vi "Sousvi2.vi"(0 "Combo Box 2":string(combo), 1 "Coffee extraction":bool) -> (2 "subarray":string[](array[string]), 3 "Numeric":i32, 4 "Array":bool[][](array[boolean]))   [LabVIEW 2022 SP3]
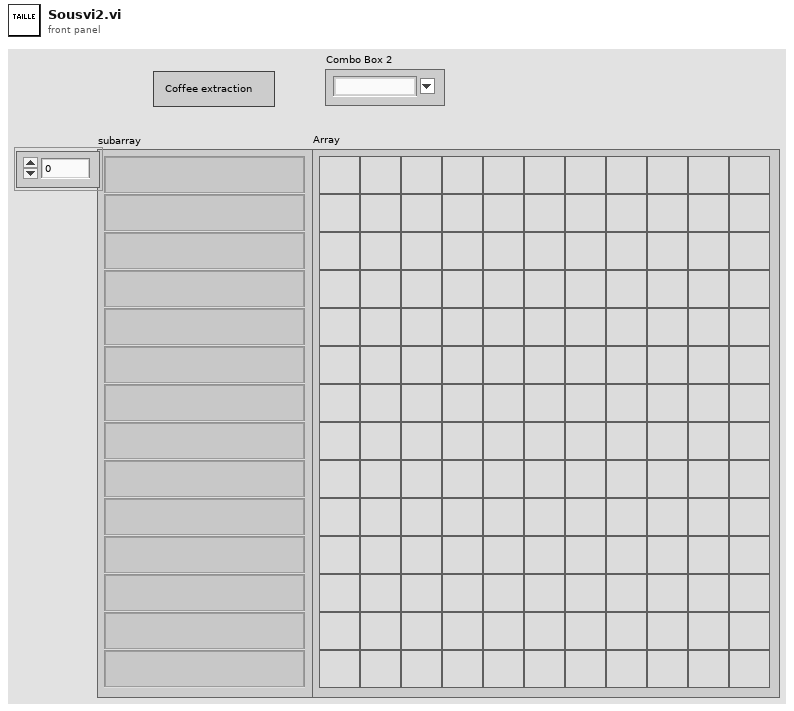
[diagram p1: front panel]
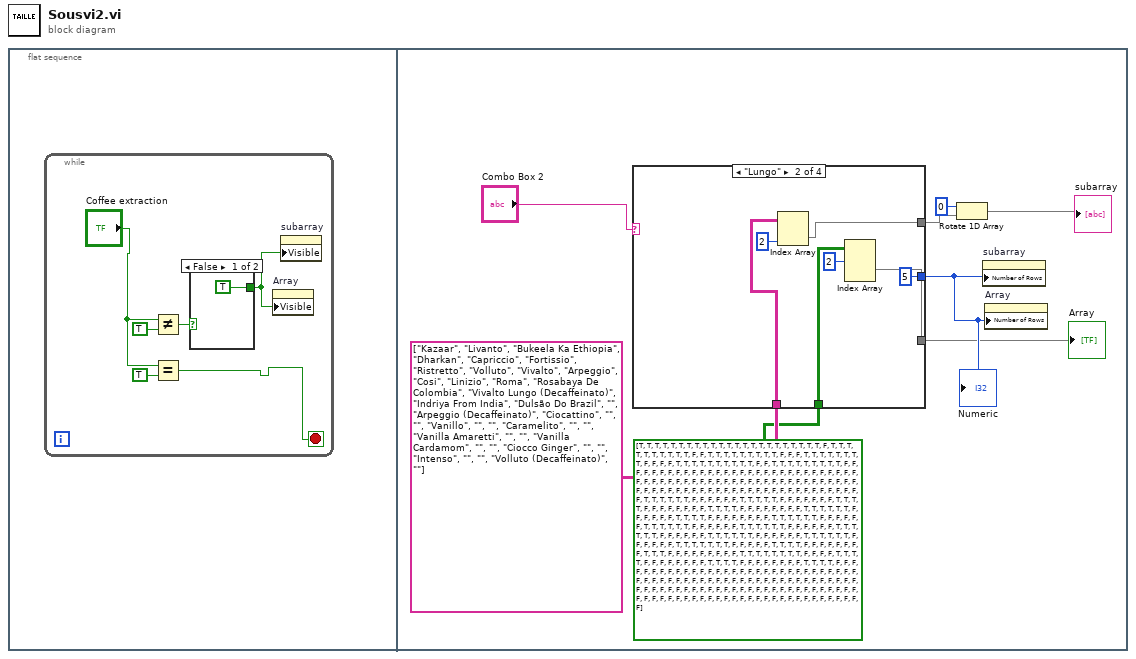
[diagram p0: block diagram]
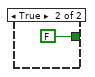
[diagram p2: hidden frame]
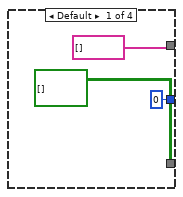
[diagram p3: hidden frame]
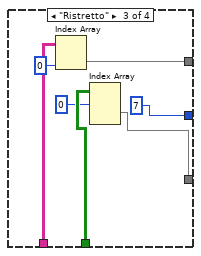
[diagram p4: hidden frame]
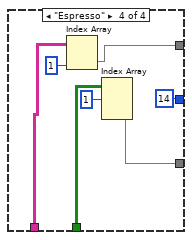
[diagram p5: hidden frame]
diagram:
  n1 = flat-sequence {
    frame #0 {
      n2 = while {
        stop <- w1 stop-if-true
        n3 = Not Equal?(x="Coffee extraction", y=TRUE) -> (x != y?=w5:bool)
        n4 = Equal?(x="Coffee extraction", y=TRUE) -> (x = y?=w1:bool)
        n5 = case shown="False" w5 {
          tunnel: [TRUE FALSE] -> w2
          frame False {
          }
          frame True {
          }
        }
        n6 = property on="Array" class="Arr (strict)"("Visible"=w2) -> ()  [unwired: 2 in, 2 out]
        n7 = property on="subarray" class="Arr (strict)"("Visible"=w2) -> ()  [unwired: 2 in, 2 out]
      }
    }
    frame #1 {
      n8 = case shown="\"Lungo\"" "Combo Box 2" {
        tunnel: string[][] [["Kazaar", "Livanto", "Bukeela Ka Ethiopia"], ["Dharkan", "Capriccio", "Fortissio"], ["Ristretto", "Volluto", "Vivalto"], ["Arpeggio", "Cosi", "Linizio"], ["Roma", "Rosabaya De Colombia", "Vivalto Lungo (Decaffeinato)"], ["Indriya From India", "Dulsão Do Brazil", ""], ["Arpeggio (Decaffeinato)", "Ciocattino", ""], ["", "Vanillo", ""], ["", "Caramelito", ""], ["", "Vanilla Amaretti", ""], ["", "Vanilla Cardamom", ""], ["", "Ciocco Ginger", ""], ["", "Intenso", ""], ["", "Volluto (Decaffeinato)", ""]] -> [_ w25 w33 w38]
        tunnel: [string[] [] ("subarray") w24 w31 w39] -> w13
        tunnel: [0 5 7 14] -> w16
        tunnel: bool[][][] [[[TRUE, TRUE, TRUE, TRUE, TRUE, TRUE, TRUE, TRUE, TRUE, TRUE, TRUE, TRUE], [TRUE, TRUE, TRUE, TRUE, TRUE, TRUE, TRUE, TRUE, TRUE, TRUE, TRUE, FALSE], [TRUE, TRUE, TRUE, TRUE, TRUE, TRUE, TRUE, TRUE, TRUE, TRUE, FALSE, FALSE], [TRUE, TRUE, TRUE, TRUE, TRUE, TRUE, TRUE, TRUE, TRUE, FALSE, FALSE, FALSE], [TRUE, TRUE, TRUE, TRUE, TRUE, TRUE, TRUE, TRUE, FALSE, FALSE, FALSE, FALSE], [TRUE, TRUE, TRUE, TRUE, TRUE, TRUE, TRUE, TRUE, TRUE, TRUE, FALSE, FALSE], [TRUE, TRUE, TRUE, TRUE, TRUE, TRUE, TRUE, TRUE, TRUE, FALSE, FALSE, FALSE], [FALSE, FALSE, FALSE, FALSE, FALSE, FALSE, FALSE, FALSE, FALSE, FALSE, FALSE, FALSE], [FALSE, FALSE, FALSE, FALSE, FALSE, FALSE, FALSE, FALSE, FALSE, FALSE, FALSE, FALSE], [FALSE, FALSE, FALSE, FALSE, FALSE, FALSE, FALSE, FALSE, FALSE, FALSE, FALSE, FALSE], [FALSE, FALSE, FALSE, FALSE, FALSE, FALSE, FALSE, FALSE, FALSE, FALSE, FALSE, FALSE], [FALSE, FALSE, FALSE, FALSE, FALSE, FALSE, FALSE, FALSE, FALSE, FALSE, FALSE, FALSE], [FALSE, FALSE, FALSE, FALSE, FALSE, FALSE, FALSE, FALSE, FALSE, FALSE, FALSE, FALSE], [FALSE, FALSE, FALSE, FALSE, FALSE, FALSE, FALSE, FALSE, FALSE, FALSE, FALSE, FALSE]], [[TRUE, TRUE, TRUE, TRUE, TRUE, TRUE, FALSE, FALSE, FALSE, FALSE, FALSE, FALSE], [TRUE, TRUE, TRUE, TRUE, TRUE, FALSE, FALSE, FALSE, FALSE, FALSE, FALSE, FALSE], [TRUE, TRUE, TRUE, TRUE, FALSE, FALSE, FALSE, FALSE, FALSE, FALSE, FALSE, FALSE], [TRUE, TRUE, TRUE, TRUE, FALSE, FALSE, FALSE, FALSE, FALSE, FALSE, FALSE, FALSE], [TRUE, TRUE, TRUE, TRUE, TRUE, TRUE, FALSE, FALSE, FALSE, FALSE, FALSE, FALSE], [TRUE, TRUE, TRUE, TRUE, FALSE, FALSE, FALSE, FALSE, FALSE, FALSE, FALSE, FALSE], [TRUE, TRUE, TRUE, TRUE, TRUE, TRUE, FALSE, FALSE, FALSE, FALSE, FALSE, FALSE], [TRUE, TRUE, TRUE, TRUE, TRUE, TRUE, FALSE, FALSE, FALSE, FALSE, FALSE, FALSE], [TRUE, TRUE, TRUE, TRUE, TRUE, TRUE, FALSE, FALSE, FALSE, FALSE, FALSE, FALSE], [TRUE, TRUE, TRUE, TRUE, TRUE, TRUE, FALSE, FALSE, FALSE, FALSE, FALSE, FALSE], [TRUE, TRUE, TRUE, TRUE, TRUE, TRUE, FALSE, FALSE, FALSE, FALSE, FALSE, FALSE], [TRUE, TRUE, TRUE, TRUE, TRUE, TRUE, FALSE, FALSE, FALSE, FALSE, FALSE, FALSE], [TRUE, TRUE, TRUE, TRUE, TRUE, TRUE, TRUE, FALSE, FALSE, FALSE, FALSE, FALSE], [TRUE, TRUE, TRUE, TRUE, FALSE, FALSE, FALSE, FALSE, FALSE, FALSE, FALSE, FALSE]], [[TRUE, TRUE, TRUE, FALSE, FALSE, FALSE, FALSE, FALSE, FALSE, FALSE, FALSE, FALSE], [TRUE, TRUE, TRUE, TRUE, TRUE, TRUE, TRUE, TRUE, FALSE, FALSE, FALSE, FALSE], [TRUE, TRUE, TRUE, TRUE, FALSE, FALSE, FALSE, FALSE, FALSE, FALSE, FALSE, FALSE], [TRUE, TRUE, TRUE, TRUE, FALSE, FALSE, FALSE, FALSE, FALSE, FALSE, FALSE, FALSE], [TRUE, TRUE, TRUE, TRUE, FALSE, FALSE, FALSE, FALSE, FALSE, FALSE, FALSE, FALSE], [FALSE, FALSE, FALSE, FALSE, FALSE, FALSE, FALSE, FALSE, FALSE, FALSE, FALSE, FALSE], [FALSE, FALSE, FALSE, FALSE, FALSE, FALSE, FALSE, FALSE, FALSE, FALSE, FALSE, FALSE], [FALSE, FALSE, FALSE, FALSE, FALSE, FALSE, FALSE, FALSE, FALSE, FALSE, FALSE, FALSE], [FALSE, FALSE, FALSE, FALSE, FALSE, FALSE, FALSE, FALSE, FALSE, FALSE, FALSE, FALSE], [FALSE, FALSE, FALSE, FALSE, FALSE, FALSE, FALSE, FALSE, FALSE, FALSE, FALSE, FALSE], [FALSE, FALSE, FALSE, FALSE, FALSE, FALSE, FALSE, FALSE, FALSE, FALSE, FALSE, FALSE], [FALSE, FALSE, FALSE, FALSE, FALSE, FALSE, FALSE, FALSE, FALSE, FALSE, FALSE, FALSE], [FALSE, FALSE, FALSE, FALSE, FALSE, FALSE, FALSE, FALSE, FALSE, FALSE, FALSE, FALSE], [FALSE, FALSE, FALSE, FALSE, FALSE, FALSE, FALSE, FALSE, FALSE, FALSE, FALSE, FALSE]]] -> [_ w22 w29 w36]
        tunnel: [bool[][] [] w21 w28 w35] -> w15
        frame Default {
        }
        frame "Lungo" {
          n9 = Index Array(array=w25, index (col)=2 ("disabled index (col)")) -> (element=w24:string[])  [unwired: 1 in]
          n10 = Index Array(array=w22, index (dim 0)=2 ("index (page)")) -> (element=w21:bool[][])  [unwired: 2 in]
        }
        frame "Ristretto" {
          n11 = Index Array(array=w33, index (col)=0 ("disabled index (col)")) -> (element=w31:string[])  [unwired: 1 in]
          n12 = Index Array(array=w29, index (dim 0)=0 ("disabled index (page)")) -> (element=w28:bool[][])  [unwired: 2 in]
        }
        frame "Espresso" {
          n13 = Index Array(array=w38, index (col)=1 ("disabled index (col)")) -> (element=w39:string[])  [unwired: 1 in]
          n14 = Index Array(array=w36, index (dim 0)=1 ("index (page)")) -> (element=w35:bool[][])  [unwired: 2 in]
        }
      }
      "Array" <- w15
      "Numeric" <- w16
      n15 = Rotate 1D Array(1:w13, 2:0 ("n")) -> (0:→"subarray":string[])
      n16 = property on="subarray" class="Arr (strict)"("Number of Rows"=w16) -> ()  [unwired: 2 in, 2 out]
      n17 = property on="Array" class="Arr (strict)"("Number of Rows"=w16) -> ()  [unwired: 2 in, 2 out]
    }
  }
